vi "Host Subfunction.vi"(8 "Input 2":dbl, 11 "Input 1":dbl) -> (3 "Output":dbl)   [LabVIEW 2018]
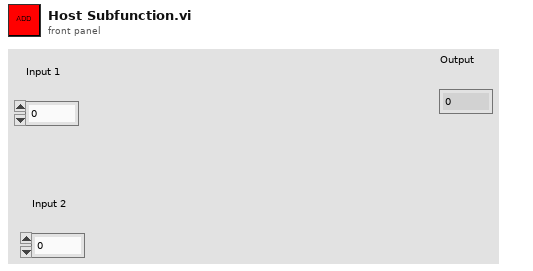
[diagram p1: front panel]
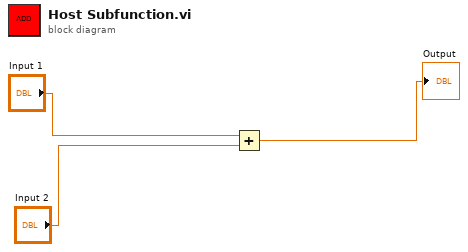
[diagram p0: block diagram]
diagram:
  n1 = Add(x="Input 1", y="Input 2") -> (x+y=→"Output":dbl)
